vi "Send Write Device IDs.vi"(7 "Message Priority (Normal)":T2=enum."Normal", 8 "error in":errorcluster, 9 "Microgrid ID":u8, 10 "Device IDs":T1[](array[typedef]), 11 "Message Enqueuer":refnum<class "Message Enqueuer.lvclass">) -> (0 "error out":errorcluster, 3 "Message Enqueuer out":refnum<class "Message Enqueuer.lvclass">)   [LabVIEW 2018, in "EMS User Interface Actor.lvlib" / "Write Device IDs Msg.lvclass"]
doc: "This VI sends the message to an actor."
uses:
  Write Device IDs Msg.lvclass
  <vilib>/ActorFramework/Message Enqueuer/Message Enqueuer.lvclass
  <vilib>/ActorFramework/Message Enqueuer/Message Priority.ctl
  <vilib>/ORNL/CSEISMIC DDS/CSEISMIC DDS Base/Data Types/Controls/DeviceID.ctl
  C:/Users/Administrator/Desktop/2018LabVIEW EMS/Dialog Actors/Devices to Load Actor/Devices to Load Messages/Return Devices to Load IDs Msg/Return Devices to Load IDs Msg.lvclass
  Dialog Actors/Devices to Load Actor/Devices to Load Messages/Return Devices to Load IDs Msg/Return Devices to Load IDs Msg.lvclass/Return Devices to Load IDs Msg.ctl
  <vilib>/ActorFramework/Message Enqueuer/Message Enqueuer.lvclass/Message Enqueuer.ctl
  <vilib>/ActorFramework/Message Enqueuer/Enqueue.vi
  Dialog Actors/Devices to Load Actor/Devices to Load Messages/Return Devices to Load IDs Msg/Return Devices to Load IDs Msg.lvclass
  C:/Program Files (x86)/National Instruments/LabVIEW 2018/vi.lib/ActorFramework/Message/Message.lvclass
  <vilib>/ActorFramework/Message Priority Queue/Priority Enqueue.vi
  <vilib>/ORNL/CSEISMIC DDS/CSEISMIC DDS Base/CSEISMIC DDS.lvclass
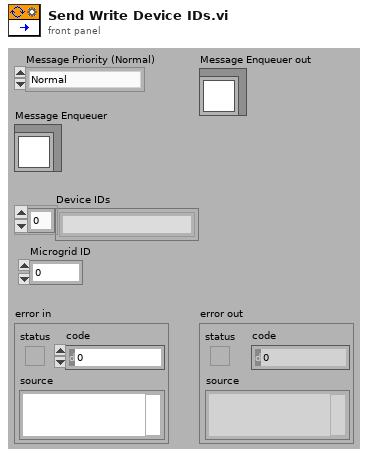
[diagram p1: front panel]
types:
  T1 = typedef "CSEISMIC DDS.lvlib/CSEISMIC DDS.lvclass/DeviceID.ctl" = string
  T2 = typedef "Actor Framework.lvlib/Message Enqueuer.lvclass/Message Priority.ctl" = enum16{"Low", "Normal", "High"}
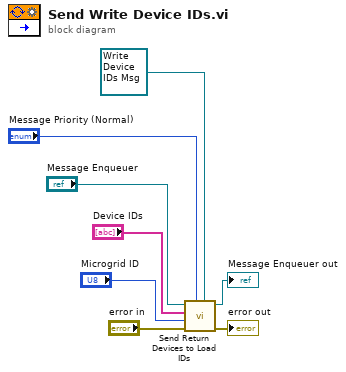
[diagram p0: block diagram]
diagram:
  n1 = call "Send Return Devices to Load IDs.vi"("Message Type"=refnum<class "Write Device IDs Msg.lvclass"> refnum ("Master Controller Core.lvlib:Write Device IDs Msg.lvclass"), "Message Priority (Normal)"="Message Priority (Normal)", "error in (no error)"="error in", "Microgrid ID"="Microgrid ID", "Device IDs"="Device IDs", "Message Enqueuer"="Message Enqueuer") -> ("error out"=→"error out":errorcluster, "Message Enqueuer out"=→"Message Enqueuer out":refnum<class "Message Enqueuer.lvclass">)  [unwired: 4 in]
